vi "pid控制.vi"(1 "kd2":dbl, 2 "kp2":dbl, 3 "当前ENC":dbl, 4 "ki2":dbl, 5 "目标ENC":dbl, 6 "ENC调节比例":dbl, 7 "kd1":dbl, 8 "ki1":dbl, 9 "kp1":dbl, 10 "当前ADC":dbl, 11 "目标ADC":dbl) -> (0 "PWM输出":dbl)   [LabVIEW 2022 SP3]
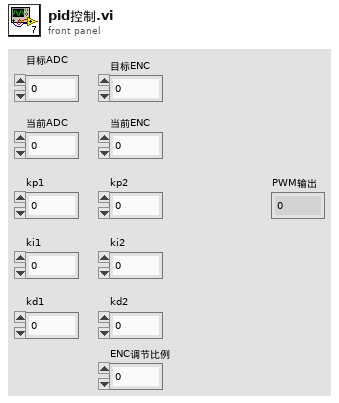
[diagram p1: front panel]
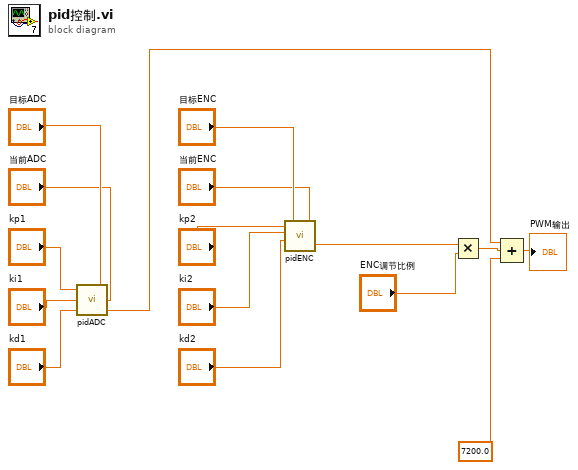
[diagram p0: block diagram]
diagram:
  n1 = call "pidADC.vi"("当前值"="当前ADC", "目标值"="目标ADC", "kd"="kd1", "ki"="ki1", "kp"="kp1") -> ("输出"=w11:dbl)
  n2 = call "pidENC.vi"("当前值"="当前ENC", "目标值"="目标ENC", "kd"="kd2", "ki"="ki2", "kp"="kp2") -> ("输出"=w3:dbl)
  n3 = Multiply(x=w3, y="ENC调节比例") -> (x*y=w1:dbl)
  n4 = Compound Arithmetic op=ADD(w11, w1, 7200.0 ("值")) -> (→"PWM输出":dbl)
